vi "(SubVI)_Control_tab_CO_Ini_Multi-Site.vi"(0 "Sti. Gal 2 AOs Ctr (Ctr2)":tag="Dev5/ctr2", 5 "Sti. Gal 2 AOs Ctr Term (PFI2)":tag="/Dev5/PFI2", 7 "AO sample rate":dbl=15000.0) -> (6 "Sti. Gal AOs Ctr Task Out":refnum<k21>, 15 "error out Ini of IO Chs":errorcluster)   [LabVIEW 2019]
uses:
  <vilib>/DAQmx/create/channels.llb/DAQmx Create Channel (CO-Pulse Generation-Frequency).vi
  <vilib>/DAQmx/configure/timing.llb/DAQmx Timing (Implicit).vi
  <resource>/objmgr/daqmx.rc
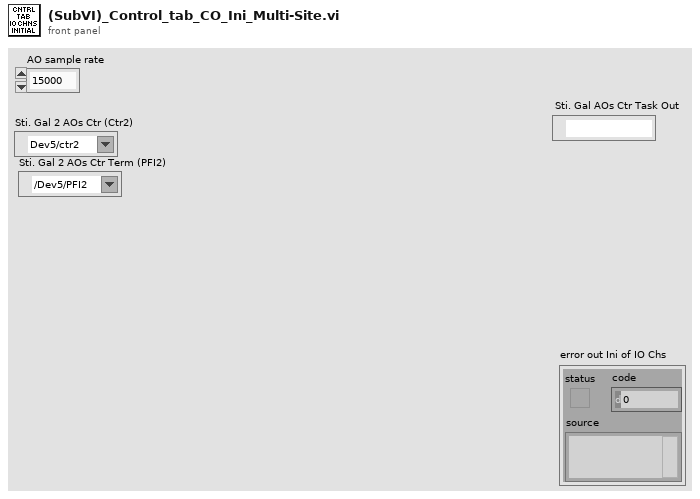
[diagram p1: front panel]
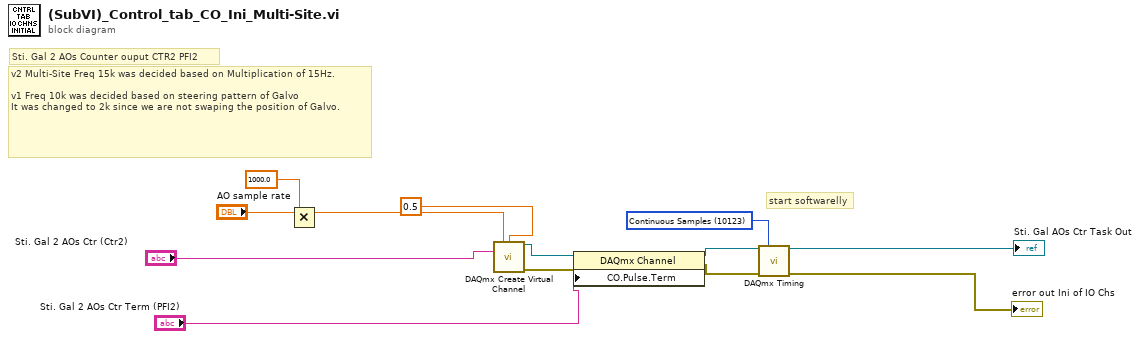
[diagram p0: block diagram]
diagram:
  w7 = 10123 items=["Finite Samples"=10178, "Continuous Samples"=10123, "Hardware Timed Single Point"=12522] ("sample mode")
  # "v2 Multi-Site Freq 15k was decided based on Multiplication of 15Hz.\n\nv1 Freq 10k was decided based on steering pattern of Galvo   \nIt was changed to 2k since we are not swaping the position of Galvo."
  # "start softwarelly"
  # "Sti. Gal 2 AOs Counter ouput CTR2 PFI2"
  n1 = Multiply(x="AO sample rate", y=1000.0) -> (x*y=w2:dbl)
  n2 = call-poly <vilib>:"DAQmx Create Virtual Channel.vi"("frequency"=w2, "duty cycle"=0.5, "counter"="Sti. Gal 2 AOs Ctr (Ctr2)") -> ("task out"=w11:refnum<k21>, "error out"=w10:errorcluster)  [unwired: 6 in, 5 out]
  n3 = property class="DAQmx Channel"(reference=w11, error in=w10, "CO.Pulse.Term"="Sti. Gal 2 AOs Ctr Term (PFI2)") -> (reference out=w9:refnum<k21>, error out=w8:errorcluster)
  n4 = call-poly <vilib>:"DAQmx Timing.vi"("task/channels in"=w9, "sample mode"=w7, "error in"=w8) -> ("task out"=→"Sti. Gal AOs Ctr Task Out":refnum<k21>, "error out"=→"error out Ini of IO Chs":errorcluster)  [unwired: 11 in]
